vi "Process Run Fault.vi"(11 "RUN Fault":u32) -> (3 "MC Fault":T1)   [LabVIEW 2014]
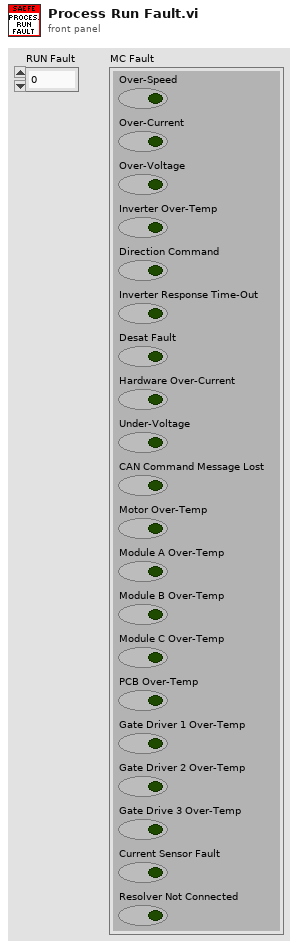
[diagram p1: front panel]
types:
  T1 = cluster{"Over-Speed":bool, "Over-Current":bool, "Over-Voltage":bool, "Inverter Over-Temp":bool, "Direction Command":bool, "Inverter Response Time-Out":bool, "Desat Fault":bool, "Hardware Over-Current":bool, "Under-Voltage":bool, "CAN Command Message Lost":bool, "Motor Over-Temp":bool, "Module A Over-Temp":bool, "Module B Over-Temp":bool, "Module C Over-Temp":bool, "PCB Over-Temp":bool, "Gate Driver 1 Over-Temp":bool, "Gate Driver 2 Over-Temp":bool, "Gate Drive 3 Over-Temp":bool, "Current Sensor Fault":bool, "Resolver Not Connected":bool}
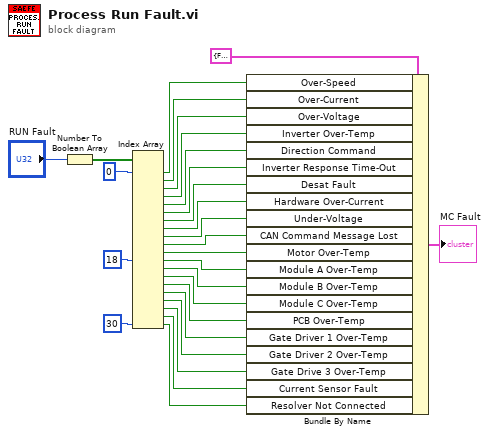
[diagram p0: block diagram]
diagram:
  n1 = Number To Boolean Array(number="RUN Fault") -> (Boolean array=w25:bool[])
  n2 = Index Array(array=w25, index #1=0 ("index"), index #12=18 ("index"), index #20=30 ("index")) -> (element #1=w22:bool, element #2=w21:bool, element #3=w20:bool, element #4=w19:bool, element #5=w18:bool, element #6=w17:bool, element #7=w16:bool, element #8=w15:bool, element #9=w14:bool, element #10=w13:bool, element #11=w12:bool, element #12=w10:bool, element #13=w9:bool, element #14=w8:bool, element #15=w7:bool, element #16=w6:bool, element #17=w5:bool, element #18=w4:bool, element #19=w3:bool, element #20=w1:bool)  [unwired: 17 in]
  n3 = Bundle By Name(cluster=T1 {"Over-Speed"=FALSE, "Over-Current"=FALSE, "Over-Voltage"=FALSE, "Inverter Over-Temp"=FALSE, "Direction Command"=FALSE, "Inverter Response Time-Out"=FALSE, "Desat Fault"=FALSE, "Hardware Over-Current"=FALSE, "Under-Voltage"=FALSE, "CAN Command Message Lost"=FALSE, "Motor Over-Temp"=FALSE, "Module A Over-Temp"=FALSE, "Module B Over-Temp"=FALSE, "Module C Over-Temp"=FALSE, "PCB Over-Temp"=FALSE, "Gate Driver 1 Over-Temp"=FALSE, "Gate Driver 2 Over-Temp"=FALSE, "Gate Drive 3 Over-Temp"=FALSE, "Current Sensor Fault"=FALSE, "Resolver Not Connected"=FALSE} ("MC Fault"), "Over-Speed"=w22, "Over-Current"=w21, "Over-Voltage"=w20, "Inverter Over-Temp"=w19, "Direction Command"=w18, "Inverter Response Time-Out"=w17, "Desat Fault"=w16, "Hardware Over-Current"=w15, "Under-Voltage"=w14, "CAN Command Message Lost"=w13, "Motor Over-Temp"=w12, "Module A Over-Temp"=w10, "Module B Over-Temp"=w9, "Module C Over-Temp"=w8, "PCB Over-Temp"=w7, "Gate Driver 1 Over-Temp"=w6, "Gate Driver 2 Over-Temp"=w5, "Gate Drive 3 Over-Temp"=w4, "Current Sensor Fault"=w3, "Resolver Not Connected"=w1) -> (→"MC Fault":T1)
